vi "getBlockStatistics.vi"(1 "Analogue Data (volts)":dbl[][](array[numeric])) -> (0 "PostProDataPerBlock":T1[][](array[typedef]))   [LabVIEW 2017]
uses:
  Controls/postProData.ctl
  Globals/measurementGlobal.vi
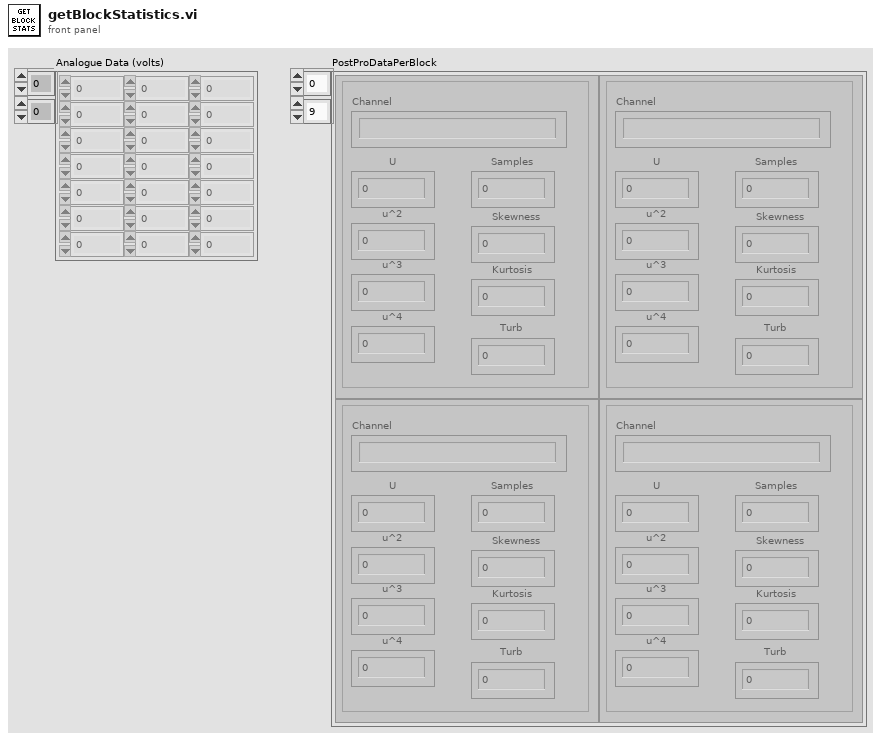
[diagram p1: front panel]
types:
  T1 = typedef "postProData.ctl" = cluster{"Channel":string, "Samples":i32, "U":dbl, "u^2":dbl, "u^3":dbl, "u^4":dbl, "Kurtosis":dbl, "Skewness":dbl, "Turb":dbl}
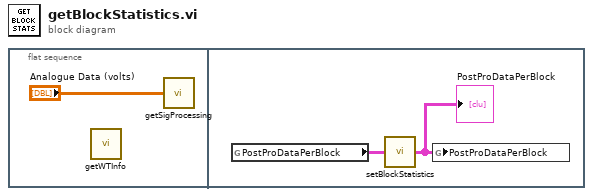
[diagram p0: block diagram]
diagram:
  n1 = flat-sequence {
    frame #0 {
      n2 = call "getWTInfo.vi"() -> ()  [unwired: 12 in]
      n3 = call "getSigProcessing.vi"("Analogue Data (volts)"="Analogue Data (volts)") -> ()  [unwired: 1 in]
    }
    frame #1 {
      n4 = global read "measurementGlobal.vi" "PostProDataPerBlock"() -> (w2:T1[][])
      n5 = call "setBlockStatistics.vi"("PostProDataPerBlock in"=w2) -> ("PostProDataPerBlock out"=w3:T1[][])
      "PostProDataPerBlock" <- w3
      n6 = global write "measurementGlobal.vi" "PostProDataPerBlock"(w3) -> ()
    }
  }
